vi "Exemple_Preprocessing_MaxAbsScaler.vi"() -> ()   [LabVIEW 2020]
uses:
  Objet/6 - Datasets Transformation/6.3 - Processing Data/MaxAbsScaler/MaxAbsScaler.lvclass
panel:
  in  "y":string[][](array[string])
  in  "X":string[][](array[string])=[["1", "-1", "2"], ["2", "0", "0"], ["0", "1", "-1"]]
  out "Data":T1
  out "error out":errorcluster
  in  "error in":errorcluster caption="entrée d'erreur"
  in  "MaxAbsScaler":cluster{"copy":bool}={"copy"=TRUE}
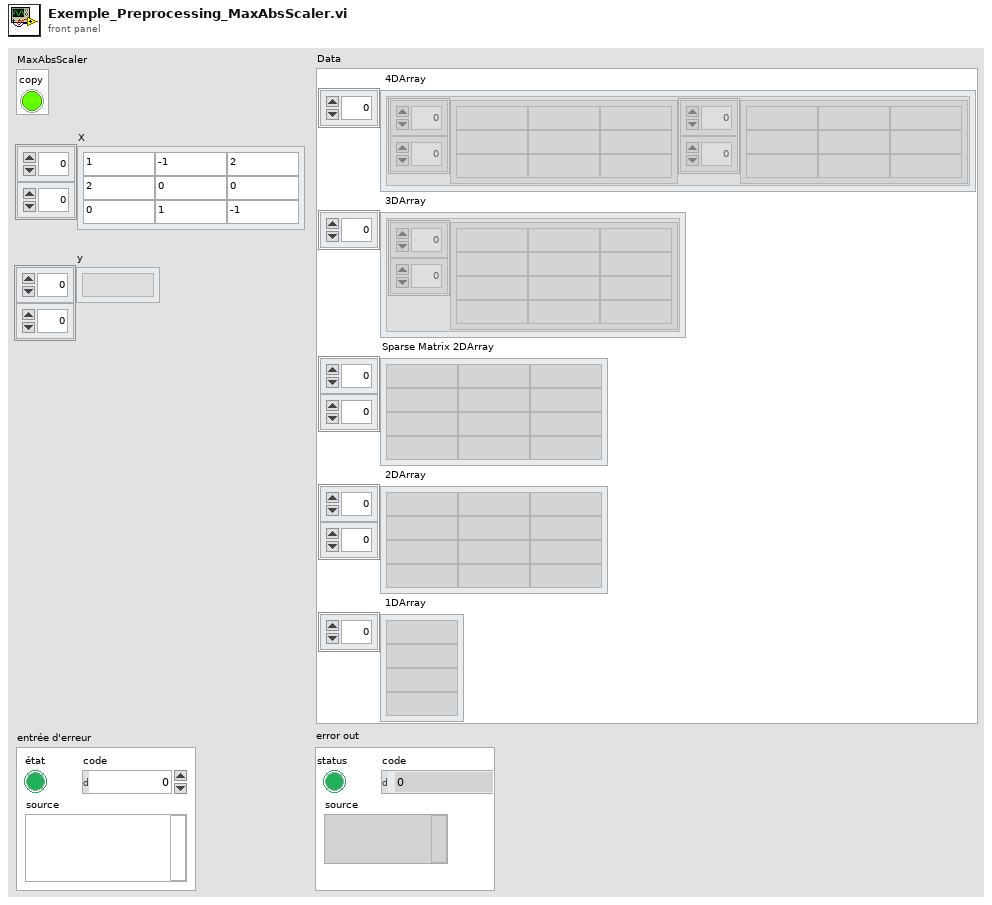
[diagram p1: front panel]
types:
  T1 = cluster{" 4DArray":cluster{"1":string[][], "2":string[][]}[], " 3DArray":cluster{"Tableau":string[][]}[], "Sparse Matrix 2DArray":string[][], " 2DArray":string[][], " 1DArray":string[]}
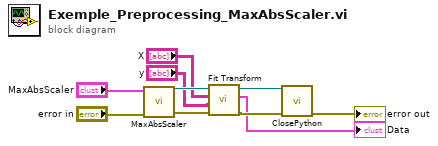
[diagram p0: block diagram]
diagram:
  n1 = call "MaxAbsScaler.vi"("error in (no error)"="error in", "MaxAbsScaler"="MaxAbsScaler") -> ("error out"=w6:errorcluster, "MaxAbsScaler.lvclass"=w9:refnum<class "MaxAbsScaler.lvclass">)  [unwired: 8 in]
  n2 = call-dynamic "Fit Transform.vi"("error in (no error)"=w6, "y"="y", "X"="X", "MaxAbsScaler.lvclass"=w9) -> ("error in (no error)"=w4:errorcluster, "Data"=→"Data":T1, "MaxAbsScaler.lvclass"=w5:refnum<class "MaxAbsScaler.lvclass">)  [unwired: 5 in]
  n3 = call-dynamic "ClosePython.vi"("error in (no error)"=w4, "Scikit-learn en entrée"=w5) -> ("error out"=→"error out":errorcluster)  [unwired: 8 in, 1 out]
